vi "Process.vi"(0 "reference in":refnum<class "Error handler.lvclass">, 5 "error in":errorcluster) -> (14 "reference out":refnum<class "Error handler.lvclass">, 19 "error out":errorcluster)   [LabVIEW 2019, in "Error handler.lvclass"]
uses:
  Error handler.lvclass
  <vilib>/Utility/SystemLogging/NI_SystemLogging.lvlib
panel:
  out "Listbox":i32[](listbox) caption="Error List"
  out "error info":errorcluster
  out "Last Command":string
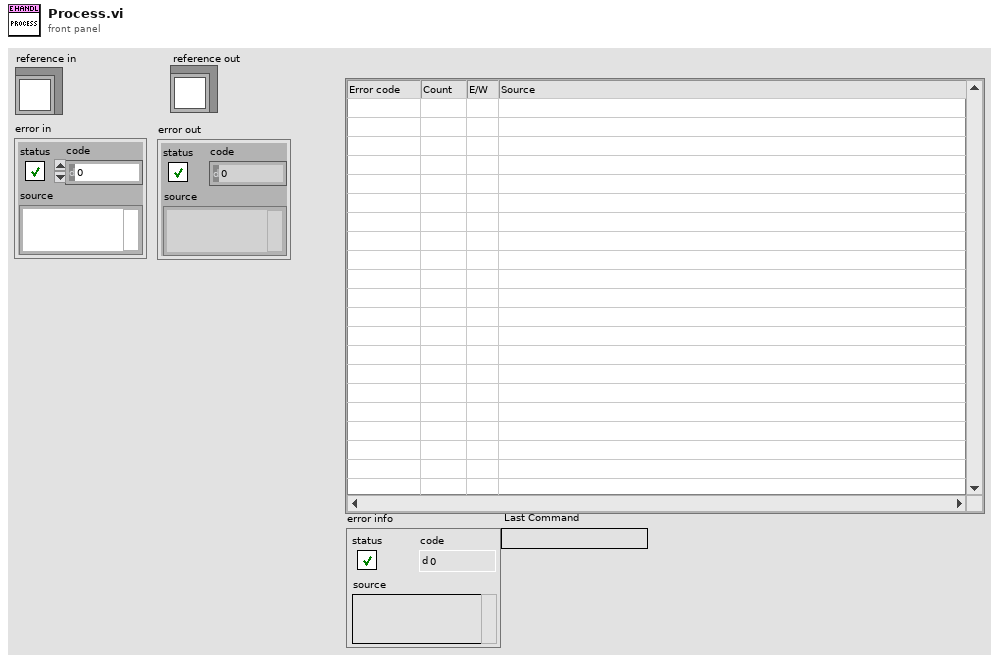
[diagram p1: front panel]
types:
  T1 = cluster{"Core":cluster{"Timeout":i32, "Events":cluster{"EventsToProcess":refnum<event-registration>}, "EventFromProcess":refnum<user-event>, "ProcessSyncQueue":refnum<queue>, "QueueFromProcess":refnum<queue>, "Command":string, "Data":variant}, "Error Map":map{i32, cluster{"error":errorcluster, "count":i32}}, "LoadFPOnError":bool, "LastReportedError":errorcluster}
  T2 = map{i32, cluster{"error":errorcluster, "count":i32}}
  T3 = enum32{"Invalid", "Standard", "Closed", "Hidden", "Minimized", "Maximized"}
  T4 = cluster{"EventsToProcess":refnum<event-registration>}
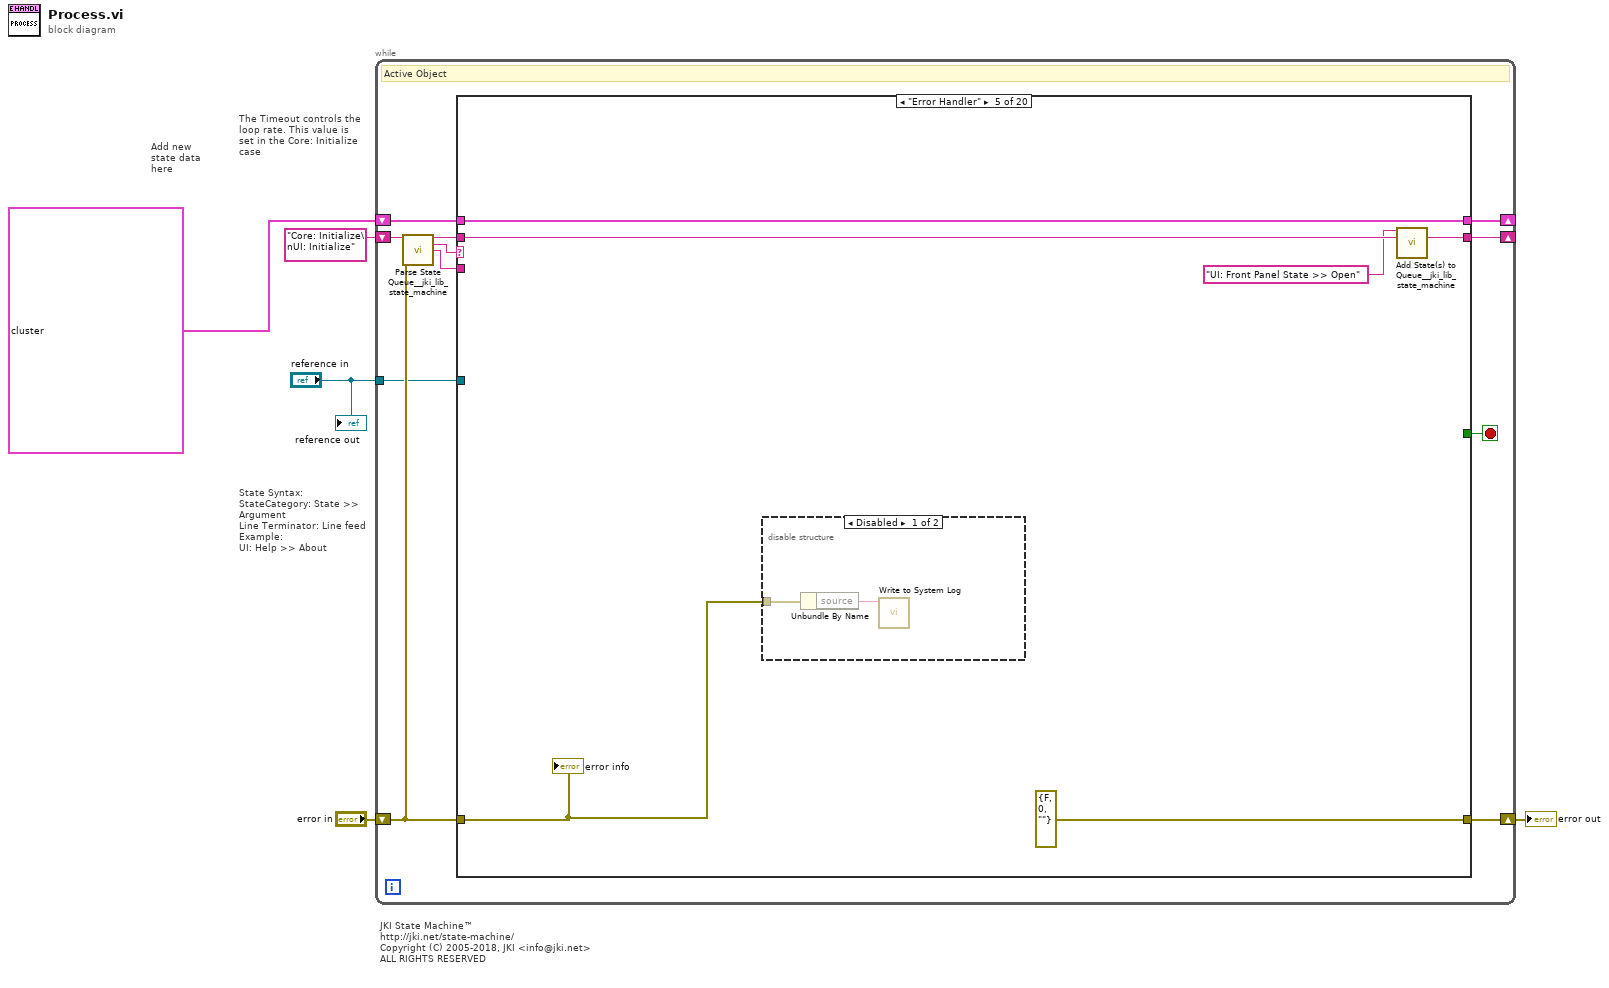
[diagram p0: block diagram]
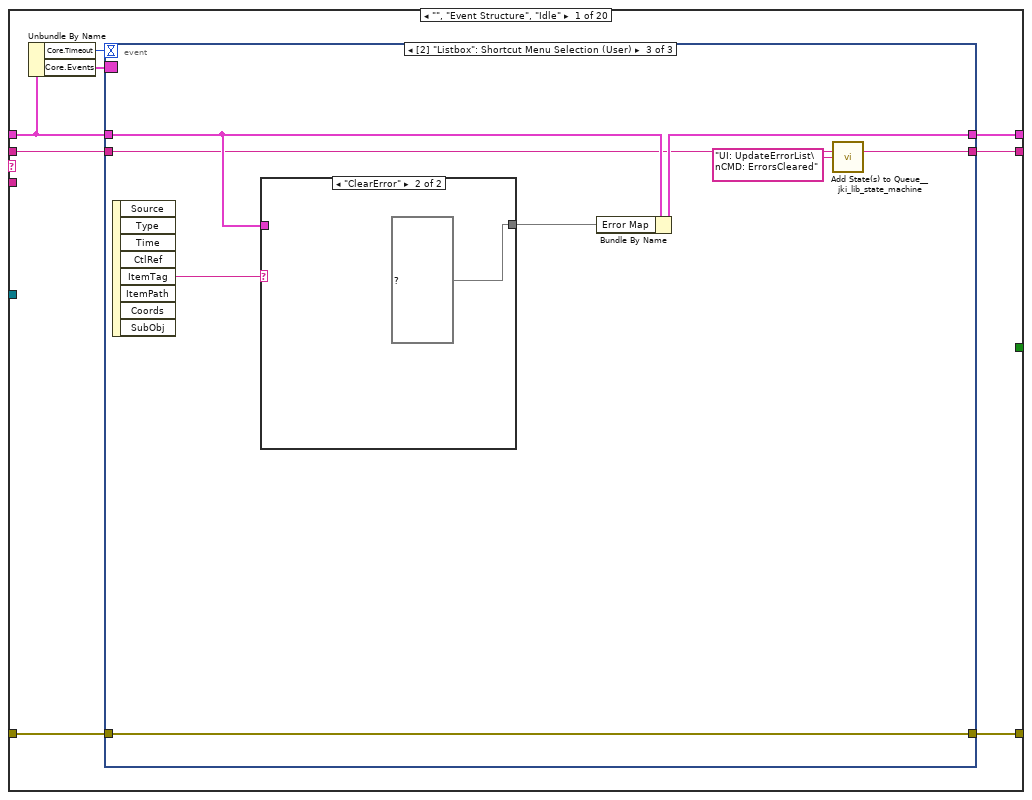
[diagram p2: hidden frame]
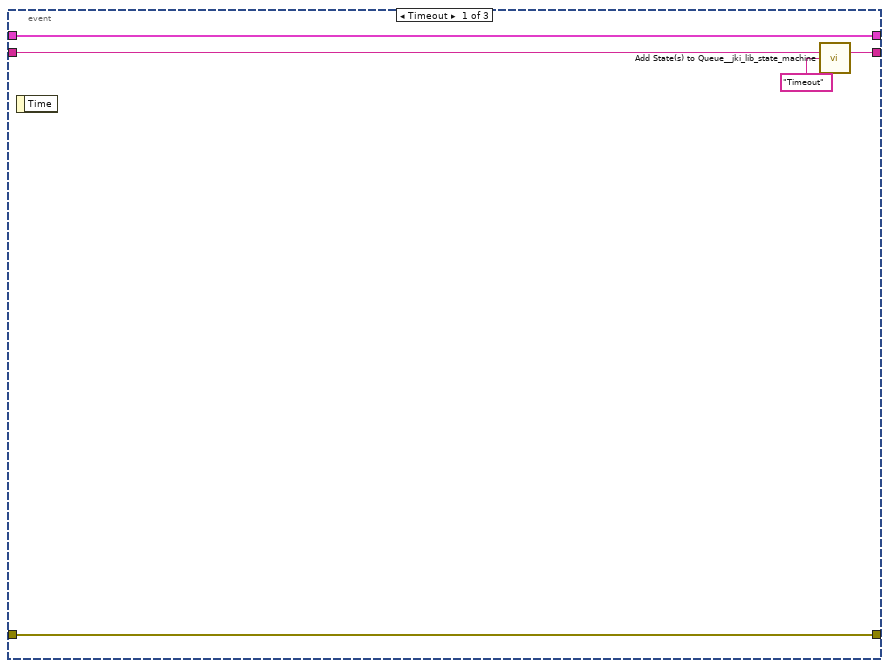
[diagram p3: hidden frame]
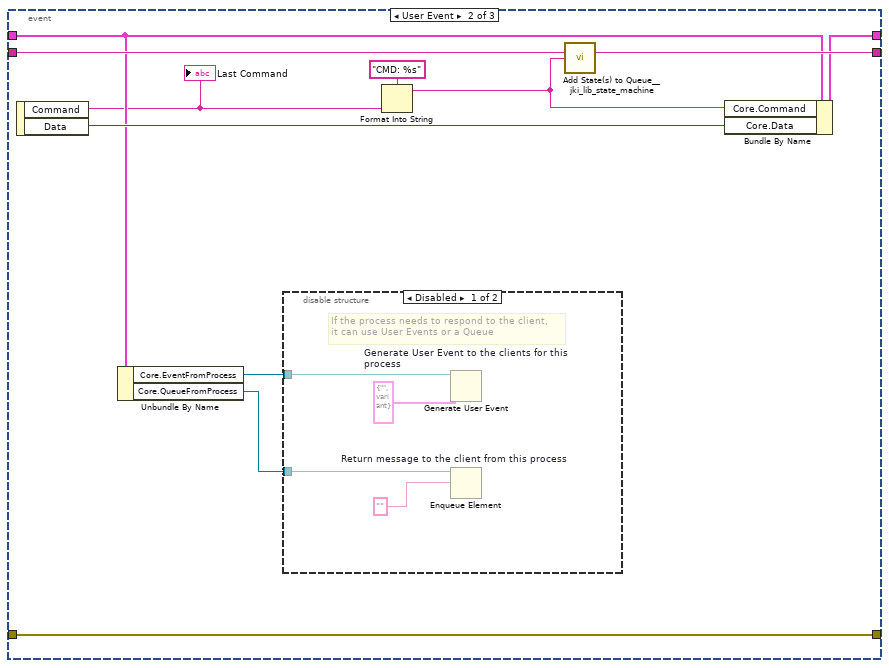
[diagram p4: hidden frame]
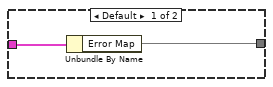
[diagram p6: hidden frame]
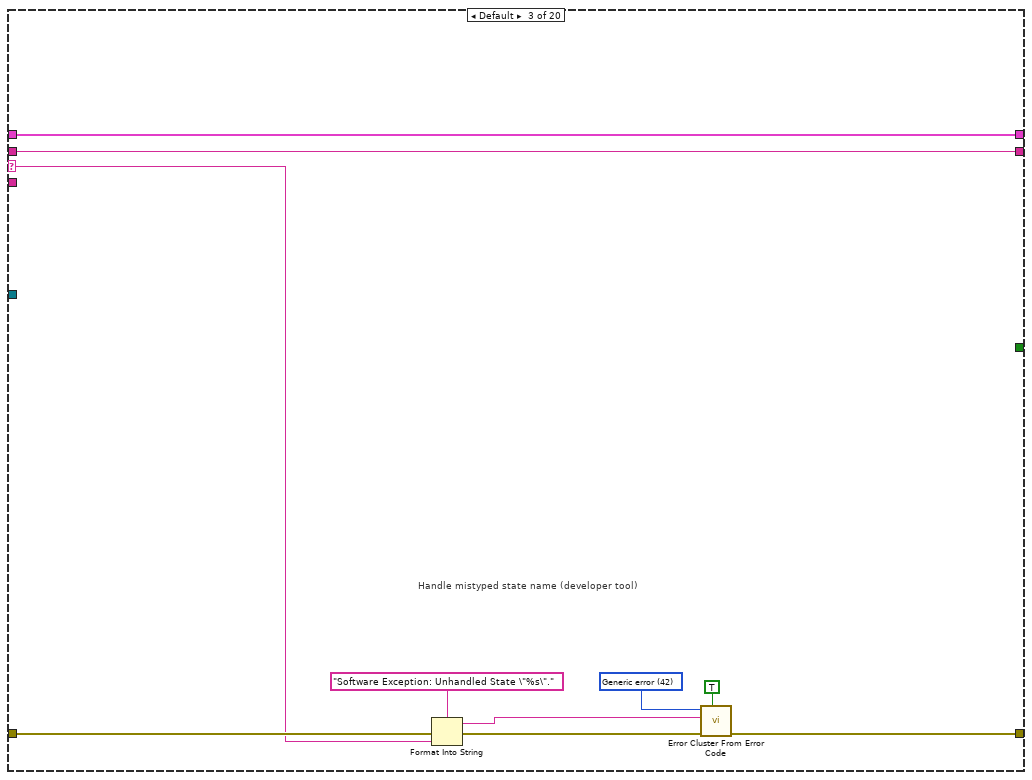
[diagram p8: hidden frame]
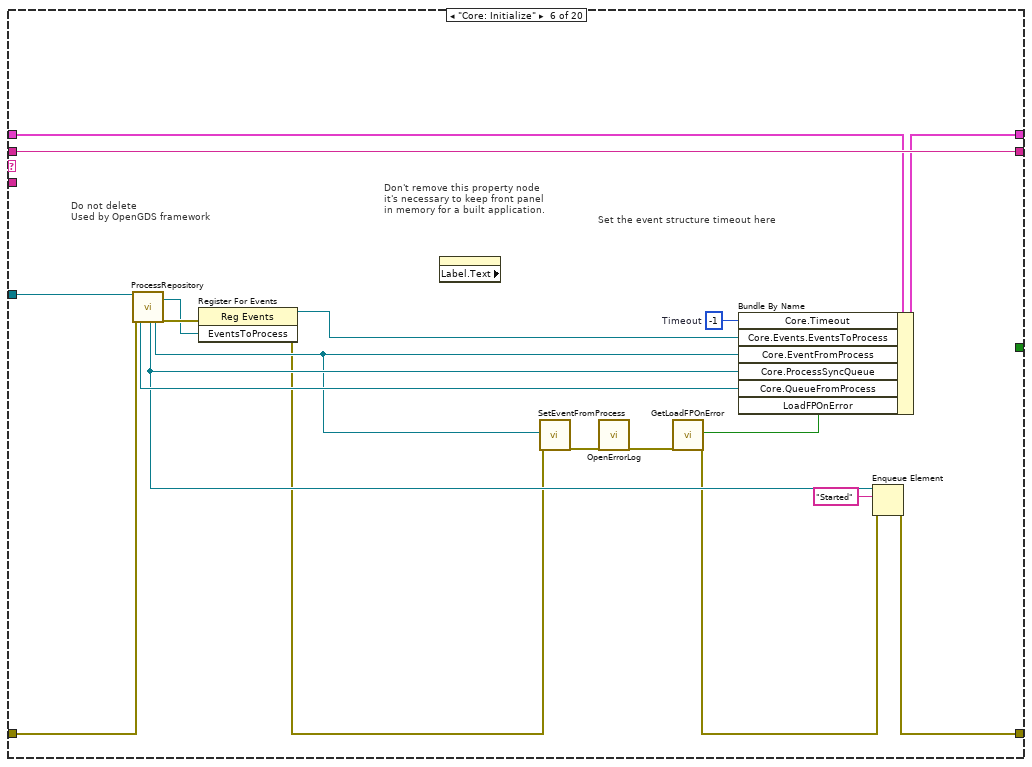
[diagram p11: hidden frame]
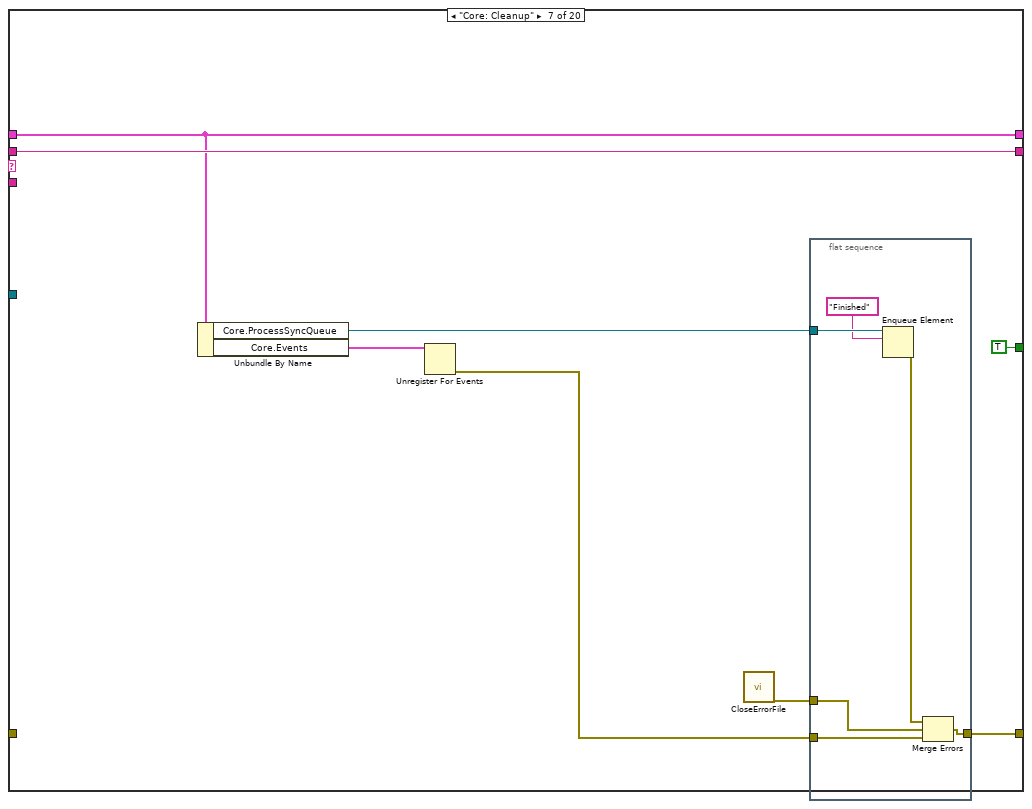
[diagram p12: hidden frame]
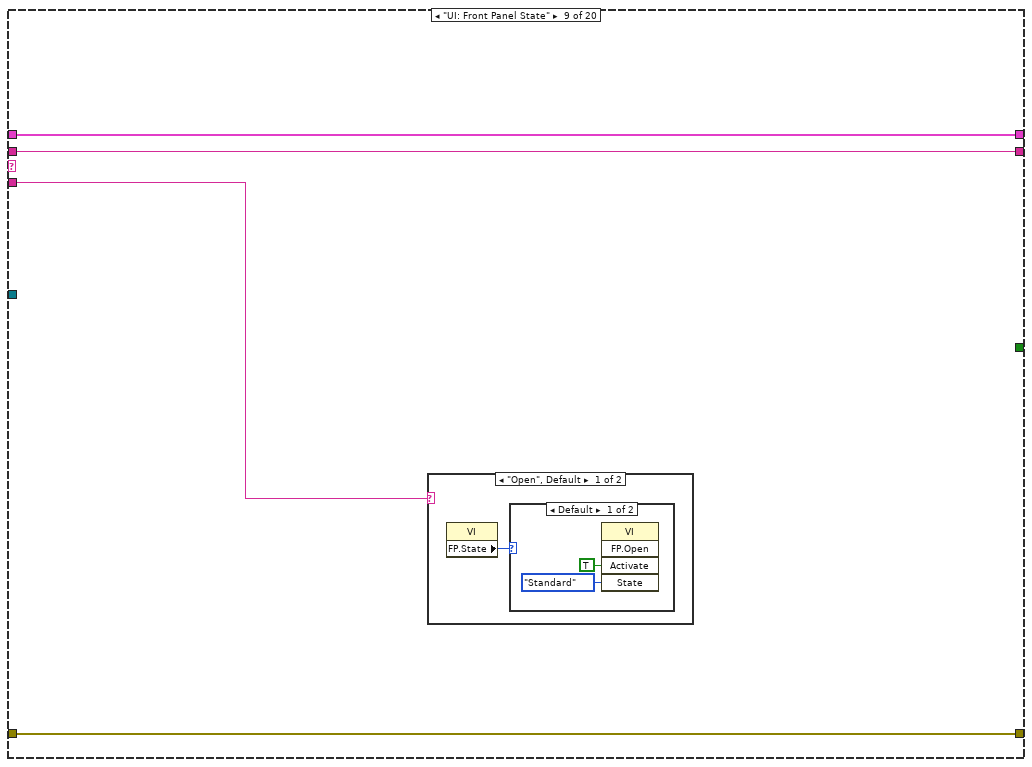
[diagram p14: hidden frame]
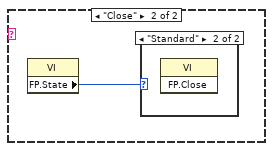
[diagram p16: hidden frame]
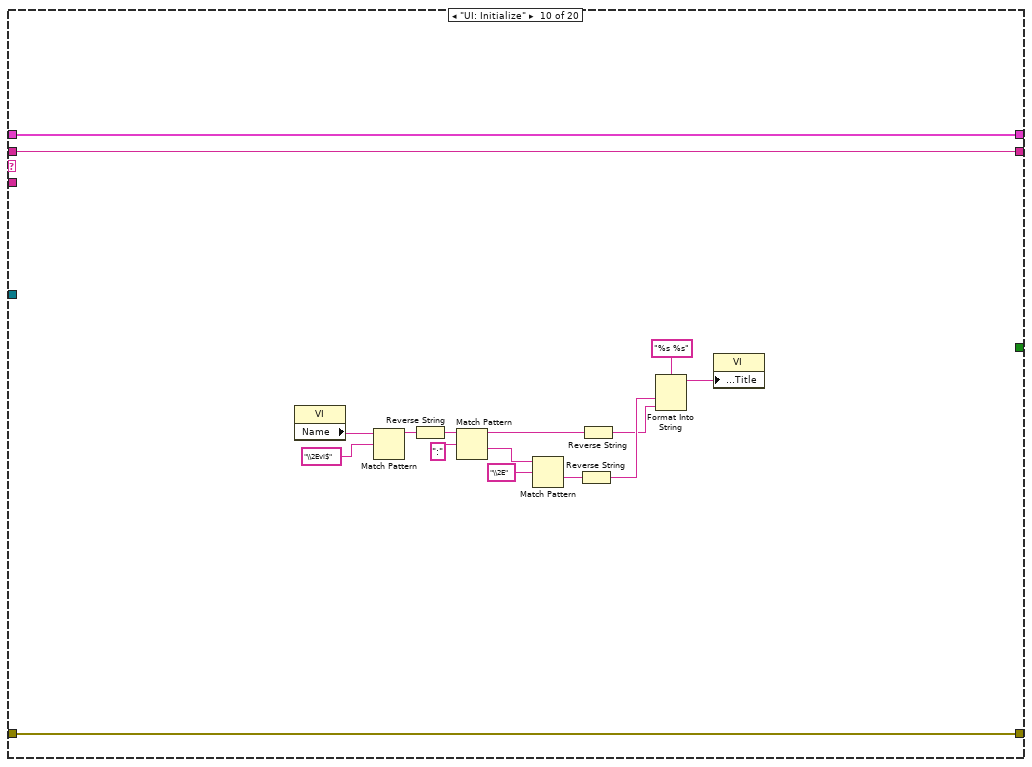
[diagram p18: hidden frame]
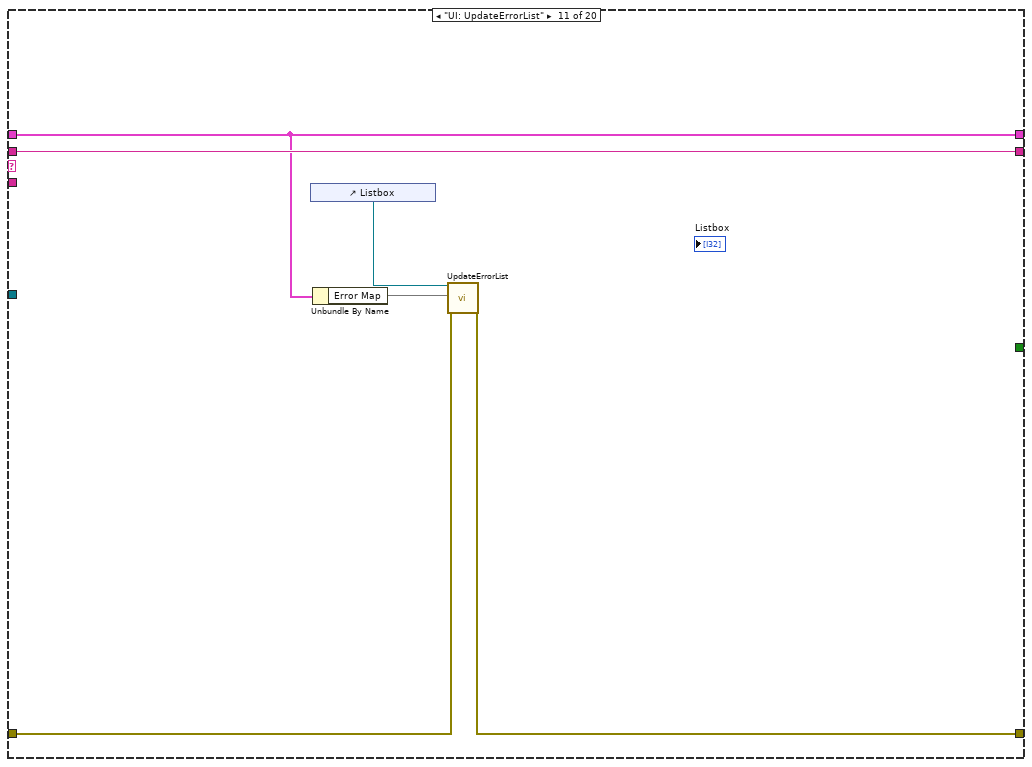
[diagram p19: hidden frame]
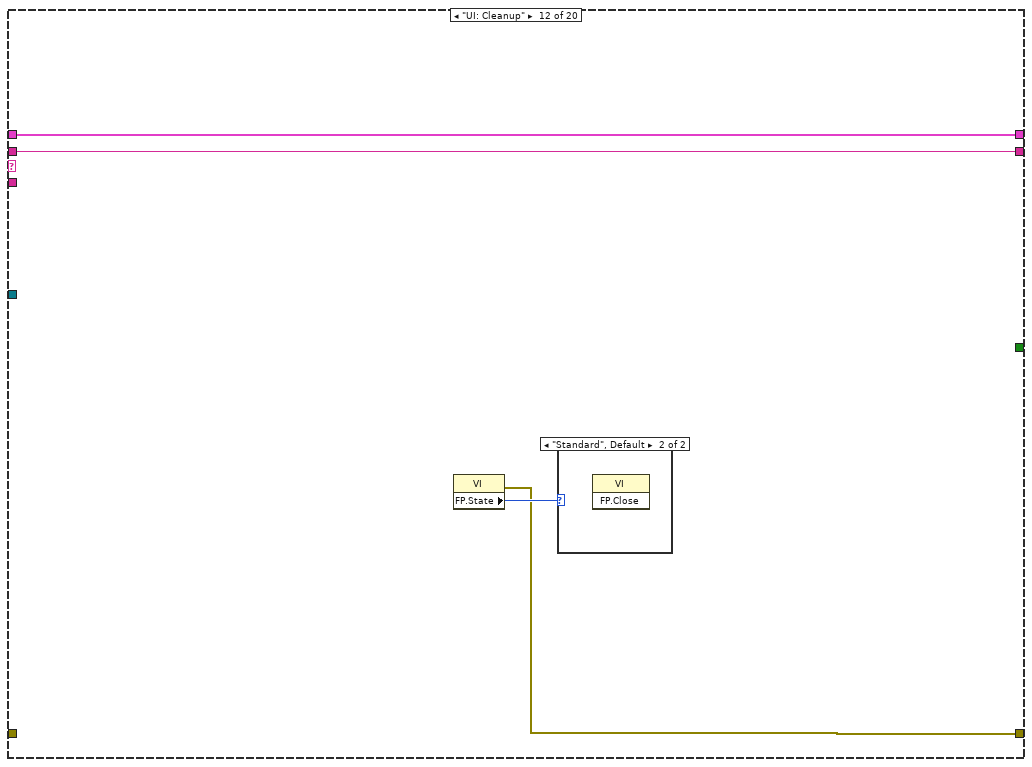
[diagram p20: hidden frame]
diagram:
  # "Add new state data here"
  # "JKI State Machine™\nhttp://jki.net/state-machine/\nCopyright (C) 2005-2018, JKI <info@jki.net>\nALL RIGHTS RESERVED"
  # "State Syntax:\nStateCategory: State >> Argument\nLine Terminator: Line feed\nExample:\nUI: Help >> About"
  # "The Timeout controls the loop rate. This value is set in the Core: Initialize case"
  n1 = while {
    shift-right: [w15] -> w4
    shift-left: "error in" -> [w16]
    shift-right: [w8] -> _
    shift-left: "Core: Initialize\nUI: Initialize" ("States Out") -> [w11]
    shift-right: [w14] -> _
    shift-left: T1 {"Core"={"Timeout"=-1, "Events"={"EventsToProcess"=refnum}, "EventFromProcess"=refnum, "ProcessSyncQueue"=refnum, "QueueFromProcess"=refnum, "Command"="", "Data"=variant}, "Error Map"={}, "LoadFPOnError"=FALSE, "LastReportedError"={"status"=FALSE, "code"=0, "source"=""}} ("LocalVariables") -> [w13]
    tunnel: "reference in" -> [w6]
    stop <- w7 stop-if-true
    # "Active Object"
    n2 = call <vilib>:"Parse State Queue__jki_lib_state_machine.vi"("State Queue"=w11, "Error In (no error)"=w16) -> ("Remaining States"=w10:string, "Current State"=w12:string, "Arguments"=w9:string)  [unwired: 11 in]
    n3 = case shown="\"Error Handler\"" w12 {
      selector: w12 -> [_ _ w59 _ _ _ _ _ _ _ _ _ _ _ _ _ _ _ _ _]
      tunnel: w16 -> [w18 w58 w61 w71 w73 w94 _ w115 w116 w139 w143 _ w152 w155 w160 w177 w189 w196 w199 w203]
      tunnel: [w19 w58 w60 w71 errorcluster {"status"=FALSE, "code"=0, "source"=""} ("error constant") w98 w102 w115 w116 w139 w144 w146 w152 w155 w169 w178 w189 w196 w199 w204] -> w15
      tunnel: [w24 w57 w68 w70 w77 w96 w103 w114 w118 w131 w142 w147 w151 w154 w171 w181 w184 w195 w198 w202] -> w14
      tunnel: w13 -> [w20 w57 w68 w70 w77 w95 w103 w114 w118 w131 w142 w147 w151 w154 w173 w181 w187 w195 w198 w202]
      tunnel: w10 -> [w22 w56 w67 w69 w76 w97 w106 w113 w119 w138 w145 w149 w150 _ w175 w182 w188 w194 w197 w205]
      tunnel: w9 -> [_ _ _ _ _ _ _ _ w117 _ _ _ _ _ _ _ _ w191 _ _]
      tunnel: [w21 w56 w67 w69 w75 w97 w106 w113 w119 w138 w145 w149 w150 "UI: Cleanup\nCore: Cleanup" ("State(s) at Back (\"\")") w166 w182 w188 w193 w197 w205] -> w8
      tunnel: [_ _ _ _ _ _ TRUE _ _ _ _ _ _ _ _ _ _ _ _ _] -> w7
      tunnel: w6 -> [_ _ _ _ _ w93 _ _ _ _ _ _ _ _ _ _ _ _ _ _]
      frame "", "Event Structure", "Idle" {
        n4 = Unbundle By Name(w20) -> ("Core.Timeout"=w17:i32, "Core.Events"=w23:T4)
        n5 = event shown="[2] \"Listbox\": Shortcut Menu Selection (User)" {
          selector: w23 -> [_ _ _]
          dyn-events: _ -> [_ _ _]
          timeout: w17 -> [_ _ _]
          tunnel: w20 -> [w29 w33 w50]
          tunnel: [w29 w38 w49] -> w24
          tunnel: [w27 w40 w47] -> w21
          tunnel: w22 -> [w28 w39 w46]
          tunnel: [w25 w34 w52] -> w19
          tunnel: w18 -> [w25 w34 w52]
          event Timeout {
            n6 = event-data() -> ()  [unwired: 1 in, 1 out]
            n7 = call <vilib>:"Add State(s) to Queue__jki_lib_state_machine.vi"("State(s) in (\"\")"=w28, "State(s) at Back (\"\")"="Timeout" ("State(s) at Back (\"\")")) -> ("States Out"=w27:string)  [unwired: 13 in]
          }
          event User Event {
            n8 = event-data() -> ("Command"=w31:string, "Data"=w37:variant)  [unwired: 1 in]
            "Last Command" <- w31
            n9 = Unbundle By Name(w33) -> ("Core.EventFromProcess"=w36:refnum<user-event>, "Core.QueueFromProcess"=w35:refnum<queue>)
            n10 = disable-structure shown="Disabled" {
              disable-tunnel: w36 -> [w44 _]
              disable-tunnel: w35 -> [w43 _]
              frame Disabled {
                # "If the process needs to respond to the client,\nit can use User Events or a Queue"
                n11 = Generate User Event "Generate User Event to the clients for this process"(user event=w44, event data cluster=cluster{"Command":string, "Data":variant} {"Command"="", "Data"=variant} ("event data")) -> ()  [unwired: 2 in, 2 out]
                n12 = Enqueue Element "Return message to the client from this process"(queue=w43, element="") -> ()  [unwired: 2 in, 3 out]
              }
              frame Enabled {
              }
            }
            n13 = Format Into String(format string="CMD: %s", w31) -> (resulting string=w30:string)  [unwired: 2 in, 1 out]
            n14 = call <vilib>:"Add State(s) to Queue__jki_lib_state_machine.vi"("State(s) in (\"\")"=w39, "State(s) at Back (\"\")"=w30) -> ("States Out"=w40:string)  [unwired: 13 in]
            n15 = Bundle By Name(cluster=w33, "Core.Command"=w30, "Core.Data"=w37) -> (w38:T1)
          }
          event "Listbox": Shortcut Menu Selection (User) {
            n16 = event-data() -> ("ItemTag"=w51:string)  [unwired: 1 in, 7 out]
            n17 = case shown="\"ClearError\"" w51 {
              tunnel: w50 -> [w54 _]
              tunnel: [w53 T2 {} ("Error Map")] -> w48
              frame Default {
                n18 = Unbundle By Name(w54) -> ("Error Map"=w53:T2)
              }
              frame "ClearError" {
              }
            }
            n19 = Bundle By Name(cluster=w50, "Error Map"=w48) -> (w49:T1)
            n20 = call <vilib>:"Add State(s) to Queue__jki_lib_state_machine.vi"("State(s) in (\"\")"=w46, "State(s) at Back (\"\")"="UI: UpdateErrorList\nCMD: ErrorsCleared" ("State(s) at Back (\"\")")) -> ("States Out"=w47:string)  [unwired: 13 in]
          }
        }
      }
      frame "---------- Core ----------" {
      }
      frame Default {
        w65 = 42 items=["No error", "Argument error", "Memory is full", "Out of zone", "End of file", "File already open", "Generic file I/O error", "File not found", "File permission error", "Disk is full", "Duplicate path", "Too many files open", "System feature not enabled", "Resource file not found", "Cannot add resource", "Resource not found", "Image not found", "Image memory error", "Pen does not exist", "Config type invalid", "Config token not found", "Config parse error", "Config memory error", "Bad external code format", "Bad external code offset", "External code not present", "Null window", "Destroy window error", "Null menu", "Print aborted", "Bad print record", "Print driver error", "Windows error during printing", "Memory error during printing", "Print dialog error", "Generic print error", "Invalid device refnum", "Device not found", "Device parameter error", "Device unit error", "Cannot open device", "Device call aborted", "Generic error", "Cancelled by user", "Object ID too low", "Object ID too high", "Object not in heap", "Unknown heap", "Unknown object (invalid DefProc)", "Unknown object (DefProc not in table)", "Message out of range", "Invalid (null) method", "Unknown message", "Manager call not supported", "Bad address", "Network operation in progress", "Network operation timed out", "Connection is busy", "Network attribute not supported", "Network error", "Address in use", "System out of memory", "Connection aborted", "Connection refused", "Not connected", "Already connected", "Connection closed", "Initialization error (interapplication manager)", "Bad occurrence", "Wait on unbound occurrence handler", "Occurrence queue overflow", "Datalog type conflict", "Unused", "Unrecognized type (interapplication manager)", "Memory corrupt", "Failed to make temporary DLL", "Old CIN version", "Drag socket not found", "Failed to load drop-object", "Failed to register OLE object", "Failed to release OLE object", "Format specifier type mismatch", "Unknown format specifier", "Too few format specifiers", "Too many format specifiers", "Scan failed", "Newer CIN version", "Error converting to variant", "Runtime menu error", "Password tampered", "Variant attribute not found", "Incompatible variant data type", "Event data is not available", "Event Store is not present", "Occurrence is not found", "Event Queue is not created", "Event info is not available", "Refnum passed is NULL", "Error retrieving Class GUID", "Error retrieving CoClass GUID", "Error retrieving TypeLib GUID.", "Bad built application magic bytes.", "Specific driver is different from the specific driver associated with the Logical Name.", "There is no session opened to the class driver.", "Max Error", "MAX - Error with config objects", "MAX - Error loading configuration", "MAX - Group not supported"]
        # "Handle mistyped state name (developer tool)"
        n21 = Format Into String(format string="Software Exception: Unhandled State \"%s\"." ("message"), error in=w61, w59) -> (resulting string=w64:string, error out=w63:errorcluster)  [unwired: 1 in]
        n22 = call <vilib>:"Error Cluster From Error Code.vi"("show call chain? (False)"=TRUE, "error in (no error)"=w63, "error message (\"\")"=w64, "error code (0)"=w65) -> ("error out"=w60:errorcluster)  [unwired: 5 in]
      }
      frame "Timeout" {
      }
      frame "Error Handler" {
        n23 = disable-structure shown="Disabled" {
          disable-tunnel: w73 -> [w79 _]
          frame Disabled {
            n24 = Unbundle By Name(w79) -> ("source"=w78:string)
            n25 = call <vilib>:"Write to System Log.vi"("message"=w78) -> ()  [unwired: 10 in, 1 out]
          }
          frame Enabled {
          }
        }
        n26 = call <vilib>:"Add State(s) to Queue__jki_lib_state_machine.vi"("State(s) in Front (\"\")"="UI: Front Panel State >> Open" ("State(s) at Back (\"\")"), "State(s) in (\"\")"=w76) -> ("States Out"=w75:string)  [unwired: 13 in]
        "error info" <- w73
      }
      frame "Core: Initialize" {
        w86 = -1  # Timeout
        # "Do not delete\nUsed by OpenGDS framework"
        # "Set the event structure timeout here"
        # "Don't remove this property node\nit's necessary to keep front panel\nin memory for a built application."
        # "Template created by VI Technologies"
        n27 = call "ProcessRepository.vi"("reference in"=w93, "Error In"=w94) -> ("QueueFromProcess"=w89:refnum<queue>, "ProcessSyncQueue"=w87:refnum<queue>, "EventFromProcess"=w85:refnum<user-event>, "EventsToProcess"=w91:refnum<user-event>, "Error Out"=w92:errorcluster)  [unwired: 10 in, 3 out]
        n28 = register-events(error in=w92, w91) -> (reference out=w90:refnum<event-registration>, error out=w84:errorcluster)  [unwired: 1 in]
        n29 = property on="reference in" class="LVClassControl (strict)" props=["Label", "Text"]() -> ()  [unwired: 2 in, 3 out]
        n30 = call "SetEventFromProcess.vi"("EventFromProcess"=w85, "Error In"=w84) -> ("Error Out"=w83:errorcluster)  [unwired: 17 in]
        n31 = call "OpenErrorLog.vi"("Error In"=w83) -> ("Error Out"=w82:errorcluster)  [unwired: 18 in]
        n32 = call "GetLoadFPOnError.vi"("Error In"=w82) -> ("LoadFPOnError"=w80:bool, "Error Out"=w81:errorcluster)  [unwired: 17 in]
        n33 = Bundle By Name(cluster=w95, "Core.Timeout"=w86, "Core.Events.EventsToProcess"=w90, "Core.EventFromProcess"=w85, "Core.ProcessSyncQueue"=w87, "Core.QueueFromProcess"=w89, "LoadFPOnError"=w80) -> (w96:T1)
        n34 = Enqueue Element(queue=w87, element="Started", error in (no error)=w81) -> (error out=w98:errorcluster)  [unwired: 1 in, 2 out]
      }
      frame "Core: Cleanup" {
        n35 = Unbundle By Name(w103) -> ("Core.ProcessSyncQueue"=w104:refnum<queue>, "Core.Events"=w101:T4)
        n36 = Unregister For Events(event registration refnum=w101) -> (error out=w100:errorcluster)  [unwired: 1 in]
        n37 = call "CloseErrorFile.vi"() -> ("Error Out"=w99:errorcluster)  [unwired: 19 in]
        n38 = flat-sequence {
          tunnel: [w112] -> w102
          tunnel: w104 -> [w111]
          tunnel: w100 -> [w110]
          tunnel: w99 -> [w107]
          frame #0 {
            n39 = Enqueue Element(queue=w111, element="Finished") -> (error out=w108:errorcluster)  [unwired: 2 in, 2 out]
            n40 = Merge Errors(w108, w107, w110) -> (w112:errorcluster)
          }
        }
      }
      frame "---------- UI ----------" {
      }
      frame "UI: Front Panel State" {
        n41 = case shown="\"Open\", Default" w117 {
          frame "Open", Default {
            n42 = property class="VI"() -> ("FP.State"=w120:T3)  [unwired: 2 in, 2 out]
            n43 = case shown="Default" w120 {
              frame Default {
                n44 = invoke class="VI" method="FP.Open"("Activate"=TRUE, "State"=T3."Standard") -> ()  [unwired: 3 in, 5 out]
              }
              frame "Standard" {
              }
            }
          }
          frame "Close" {
            n45 = property class="VI"() -> ("FP.State"=w123:T3)  [unwired: 2 in, 2 out]
            n46 = case shown="\"Standard\"" w123 {
              frame Default {
              }
              frame "Standard" {
                n47 = invoke class="VI" method="FP.Close"() -> ()  [unwired: 3 in, 3 out]
              }
            }
          }
        }
      }
      frame "UI: Initialize" {
        n48 = property class="VI"() -> ("Name"=w137:string)  [unwired: 2 in, 2 out]
        n49 = Match Pattern(string=w137, regular expression="\\2Evi$") -> (before substring=w135:string)  [unwired: 1 in, 3 out]
        n50 = Reverse String(1:w135) -> (0:w134:string)
        n51 = Match Pattern(string=w134, regular expression=":") -> (before substring=w132:string, after substring=w130:string)  [unwired: 1 in, 2 out]
        n52 = Match Pattern(string=w130, regular expression="\\2E") -> (after substring=w128:string)  [unwired: 1 in, 3 out]
        n53 = Reverse String(1:w128) -> (0:w127:string)
        n54 = Reverse String(1:w132) -> (0:w126:string)
        n55 = Format Into String(format string="%s %s", w127, w126) -> (resulting string=w125:string)  [unwired: 2 in, 1 out]
        n56 = property class="VI"("Front Panel.Title"=w125) -> ()  [unwired: 2 in, 2 out]
      }
      frame "UI: UpdateErrorList" {
        n57 = control-ref of="Listbox"() -> (w140:refnum<vi>)
        n58 = Unbundle By Name(w142) -> ("Error Map"=w141:T2)
        n59 = call "UpdateErrorList.vi"("tree listbox"=w140, "Error Map"=w141, "error in"=w143) -> ("error out"=w144:errorcluster)  [unwired: 16 in]
      }
      frame "UI: Cleanup" {
        n60 = property class="VI"() -> (error out=w146:errorcluster, "FP.State"=w148:T3)  [unwired: 2 in, 1 out]
        n61 = case shown="\"Standard\", Default" w148 {
          frame "Closed" {
          }
          frame "Standard", Default {
            n62 = invoke class="VI" method="FP.Close"() -> ()  [unwired: 3 in, 3 out]
          }
        }
      }
      frame "---------- CMD ----------" {
      }
      frame "CMD: Exit" {
      }
      frame "CMD: ReportError" {
        n63 = Unbundle By Name(w173) -> ("Core.Data"=w156:variant, "LoadFPOnError"=w167:bool, "Core.EventFromProcess"=w159:refnum<user-event>)
        n64 = Variant To Data(type=errorcluster {"status"=FALSE, "code"=0, "source"=""} ("error in"), Variant=w156) -> (data=w168:errorcluster)  [unwired: 1 in, 1 out]
        n65 = Bundle By Name(cluster=cluster{"Command":string, "Data":variant} {"Command"="Error occured", "Data"=variant} ("event data"), "Data"=w156) -> (w157:cluster{"Command":string, "Data":variant})
        n66 = Select(t="UI: Front Panel State >> Open", s=w167, f="" ("State(s) at Back (\"\")")) -> (s? t:f=w163:string)
        n67 = Unbundle By Name(w173) -> ("Error Map"=w172:T2)
        n68 = Generate User Event(user event=w159, event data cluster=w157, error in=w160) -> (error out=w161:errorcluster)  [unwired: 1 in, 1 out]
        n69 = call "AddErrorToMap.vi"("Error Map in"=w172, "Error reported"=w168, "Error In"=w161) -> ("Error Map out"=w170:T2, "Error Out"=w169:errorcluster)  [unwired: 15 in]
        n70 = Bundle By Name(cluster=w173, "Error Map"=w170, "LastReportedError"=w168) -> (w171:T1)
        n71 = call <vilib>:"Add State(s) to Queue__JKI_lib_State_Machine.vi"("State(s) in (\"\")"=w175, "State(s) at Back (\"\")"="UI: UpdateErrorList\nError: LogReportedError" ("State(s) at Back (\"\")")) -> ("States Out"=w165:string)  [unwired: 13 in]
        n72 = call <vilib>:"Add State(s) to Queue__JKI_lib_State_Machine.vi"("State(s) in (\"\")"=w165, "State(s) at Back (\"\")"=w163) -> ("States Out"=w166:string)  [unwired: 13 in]
      }
      frame "CMD: ErrorsCleared" {
        n73 = Unbundle By Name(w181) -> ("Core.EventFromProcess"=w180:refnum<user-event>)
        n74 = Generate User Event(user event=w180, event data cluster=cluster{"Command":string, "Data":variant} {"Command"="Errors cleared", "Data"=variant} ("event data"), error in=w177) -> (error out=w178:errorcluster)  [unwired: 1 in, 1 out]
      }
      frame "CMD: OpenProcessOnError" {
        n75 = Unbundle By Name(w187) -> ("Core.Data"=w186:variant)
        n76 = Variant To Data(type=FALSE, Variant=w186) -> (data=w183:bool)  [unwired: 1 in, 1 out]
        n77 = Bundle By Name(cluster=w187, "LoadFPOnError"=w183) -> (w184:T1)
      }
      frame "CMD: Front Panel State" {
        n78 = Format Into String(format string="UI: Front Panel State>>%s" ("string"), w191) -> (resulting string=w190:string)  [unwired: 2 in, 1 out]
        n79 = call <vilib>:"Add State(s) to Queue__jki_lib_state_machine.vi"("State(s) in (\"\")"=w194, "State(s) at Back (\"\")"=w190) -> ("States Out"=w193:string)  [unwired: 13 in]
      }
      frame "---------- Error ----------" {
      }
      frame "Error: LogReportedError" {
        n80 = Unbundle By Name(w202) -> ("Error Map"=w200:T2, "LastReportedError"=w201:errorcluster)
        n81 = call "LogError.vi"("Error Map"=w200, "LastReportedError"=w201, "error in"=w203) -> ("error out"=w204:errorcluster)  [unwired: 16 in]
      }
    }
  }
  "error out" <- w4
  "reference out" <- "reference in"
